vi "Move Core.vi"(6 "Relative?":bool, 8 "error in (no error)":errorcluster, 9 "Raw-Position":dbl, 10 "AxisNumber":u8, 11 "CS++Nanotec in":refnum<class "CS++Nanotec.lvclass">) -> (0 "error out":errorcluster, 3 "CS++Nanotec out":refnum<class "CS++Nanotec.lvclass">)   [LabVIEW 2015, in "CS++Nanotec.lvlib" / "CS++Nanotec.lvclass"]
doc: "Starts an absolute or relative movment of an axis."
uses:
  CS++Nanotec.lvclass
  CS++Nanotec.lvclass/CS++Nanotec.ctl
  instr.lib/NanotecSMCPD/NanotecSMCPDDriver.lvlib
  CSPP_DeviceBase/CS++Motor/CS++Motor.lvclass
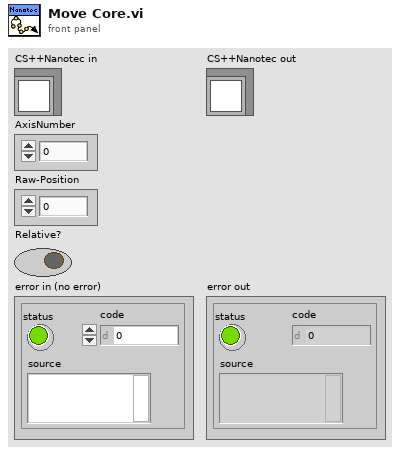
[diagram p1: front panel]
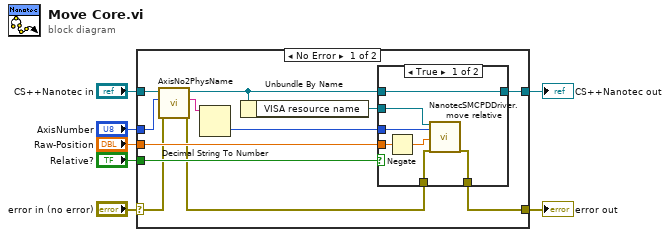
[diagram p0: block diagram]
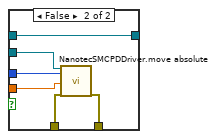
[diagram p2: hidden frame]
diagram:
  n1 = case shown="No Error" "error in (no error)" {
    selector: "error in (no error)" -> [w10 w33]
    tunnel: "CS++Nanotec in" -> [w12 w34]
    tunnel: [w18 w33] -> w5
    tunnel: "AxisNumber" -> [w13 _]
    tunnel: "Raw-Position" -> [w17 _]
    tunnel: [w16 w34] -> w2
    tunnel: "Relative?" -> [w15 _]
    frame No Error {
      n2 = call "AxisNo2PhysName.vi"("error in (no error)"=w10, "AxisNumber"=w13, "CS++Motor in"=w12) -> ("error out"=w9:errorcluster, "PhysicalChannelName"=w14:string, "CS++Motor out"=w11:refnum<class "CS++Nanotec.lvclass">)  [unwired: 6 in]
      n3 = Decimal String To Number(string=w14) -> (number=w8:i32)  [unwired: 2 in, 1 out]
      n4 = Unbundle By Name(w11) -> ("VISA resource name"=w19:refnum<visa-resource-name>)
      n5 = case shown="True" w15 {
        tunnel: w19 -> [w26 w32]
        tunnel: w9 -> [w25 w31]
        tunnel: [w24 w30] -> w18
        tunnel: w8 -> [w23 w29]
        tunnel: w17 -> [w22 w28]
        tunnel: [w21 w27] -> w16
        tunnel: w11 -> [w21 w27]
        frame True {
          n6 = Negate(x=w22) -> (-x=w20:dbl)
          n7 = call "NanotecSMCPDDriver.move relative.vi"("VISA resource name"=w26, "contollerID"=w23, "nOfSteps [uSteps]"=w20, "error in (no error)"=w25) -> ("error out"=w24:errorcluster)  [unwired: 13 in, 2 out]
        }
        frame False {
          n8 = call "NanotecSMCPDDriver.move absolute.vi"("VISA resource name"=w32, "contollerID"=w29, "nOfSteps [uSteps]"=w28, "error in (no error)"=w31) -> ("error out"=w30:errorcluster)  [unwired: 13 in, 2 out]
        }
      }
    }
    frame Error {
    }
  }
  "error out" <- w5
  "CS++Nanotec out" <- w2
